vi "Query Sweep Frequency.vi"(7 "Sweep Frequency":T1, 8 "error in (no error)":errorcluster, 10 "Channel (0: Channel 1)":T2 items=["Channel 1", "Channel 2"], 11 "VISA resource name":refnum<visa-resource-name>) -> (0 "error out":errorcluster, 1 "frequency":dbl[unit], 3 "VISA resource name out":refnum<visa-resource-name>)   [LabVIEW 2023, in "Tektronix AFG 3000 Series.lvlib"]
doc: "Queries the specified sweep frequency (center, span, start, or stop) of a Tektronix AFG 3000 series function generator. Used in sweep mode."
uses:
  Tektronix AFG 3000 Series.lvlib
  controls.llb/Channel.ctl
  controls.llb/Sweep Frequency.ctl
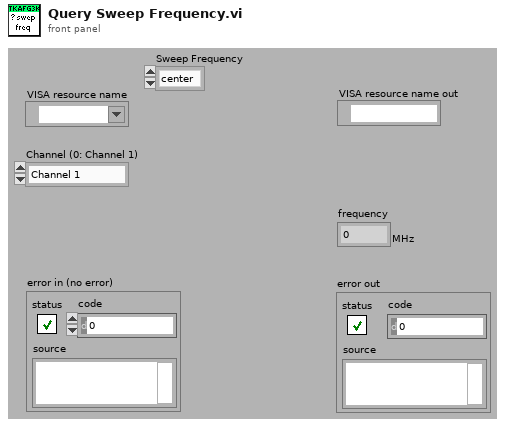
[diagram p1: front panel]
types:
  T1 = typedef "Sweep Frequency.ctl" = enum16{"center", "span", "start", "stop"}
  T2 = typedef "Channel.ctl" = u16
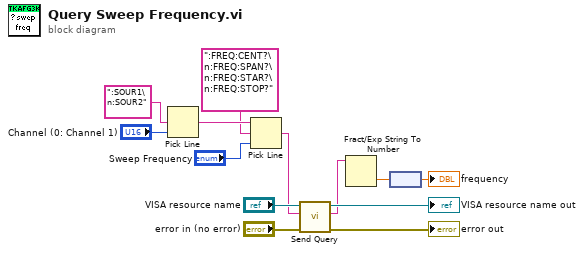
[diagram p0: block diagram]
diagram:
  n1 = Pick Line(multi-line string=":SOUR1\n:SOUR2", line index="Channel (0: Channel 1)") -> (output string=w4:string)  [unwired: 1 out]
  n2 = Pick Line(string ("")=w4, multi-line string=":FREQ:CENT?\n:FREQ:SPAN?\n:FREQ:STAR?\n:FREQ:STOP?" ("format string"), line index="Sweep Frequency") -> (output string=w2:string)
  n3 = call "Send Query.vi"("error in (no error)"="error in (no error)", "write buffer"=w2, "VISA resource name"="VISA resource name") -> ("error out"=→"error out":errorcluster, "read buffer"=w7:string, "VISA resource name out"=→"VISA resource name out":refnum<visa-resource-name>)  [unwired: 1 in, 5 out]
  n4 = Fract/Exp String To Number(string=w7) -> (number=w6:dbl)  [unwired: 4 out]
  n5 = node(w6) -> (→"frequency":dbl[unit])
